vi "On File Close.vi"(8 "error in (no error)":errorcluster, 10 "Path":path, 11 "File Close Event Registrations in":T1[](array[typedef])) -> (0 "error out":errorcluster, 3 "File Close Event Registrations out":T1[](array[typedef]))   [LabVIEW 2015, in "Segmented Log.lvclass"]
uses:
  Segmented Log.lvclass
  File Close Event Registration.ctl
  File Close Event Data.ctl
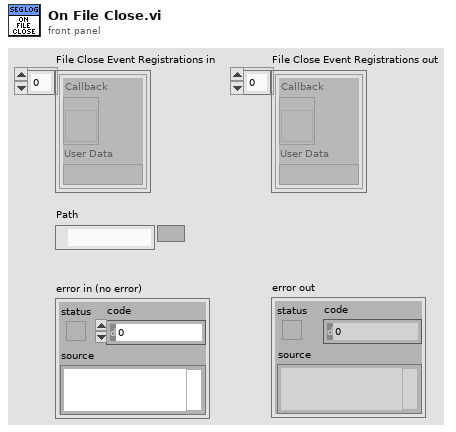
[diagram p1: front panel]
types:
  T1 = typedef "Segmented Log.lvclass/File Close Event Registration.ctl" = cluster{"Callback":refnum<vi>, "User Data":variant}
  T2 = typedef "Segmented Log.lvclass/File Close Event Data.ctl" = cluster{"File Path":path, "User Data":variant}
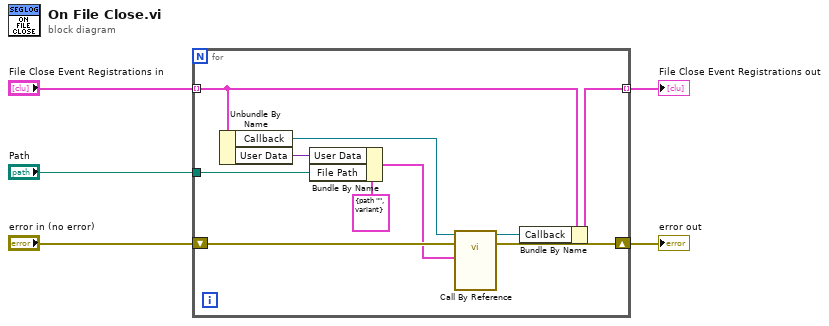
[diagram p0: block diagram]
diagram:
  n1 = for {
    tunnel: "File Close Event Registrations in" -> [w12] mode=indexing
    shift-right: [w13] -> w2
    shift-left: "error in (no error)" -> [w15]
    tunnel: [w11] -> w4 mode=indexing
    tunnel: "Path" -> [w6]
    n2 = Unbundle By Name(w12) -> ("Callback"=w14:refnum<vi>, "User Data"=w8:variant)
    n3 = Bundle By Name(cluster=T2 {"File Path"=path "", "User Data"=variant} ("File Close Event Data"), "User Data"=w8, "File Path"=w6) -> (w9:T2)
    n4 = call-by-ref "?"(reference=w14, error in=w15, "File Open Event Data"=w9) -> (reference out=w10:refnum<vi>, error out=w13:errorcluster)  [unwired: 11 in]
    n5 = Bundle By Name(cluster=w12, "Callback"=w10) -> (w11:T1)
  }
  "error out" <- w2
  "File Close Event Registrations out" <- w4
